vi "QuadRotor_Monitoring_LV3.vi"() -> ()   [LabVIEW 2015]
uses:
  <vilib>/Instr/_visa.llb/VISA Set IO Buffer Mask.ctl
  <vilib>/Instr/_visa.llb/VISA Configure Serial Port (Instr).vi
panel:
  out "GPS_Distance_T_G":dbl(slide) scale=0.0..200.0
  out "GPS_Distance__H_G":dbl(slide) scale=0.0..200.0
  out "GPS_Speed_Gaud":ext(knob) scale=0.0..80.0
  out "GPS_Distance_Transport":ext format="%#_3g"
  out "GPS_Distance_Home":ext format="%#_3g"
  out "GPS_LON_TRANSPORT":ext format="%#.7f"
  out "GPS_LAT_TRANSPORT":ext format="%#.7f"
  out "GPS_LON_HOME":ext format="%#.7f"
  out "GPS_LAT_HOME":ext format="%#.7f"
  out "Distance_R":dbl(slide)
  out "Distance_B":dbl(slide)
  out "Distance_F":dbl(slide) scale=0.0..800.0
  out "Distance_L":dbl(slide) scale=0.0..800.0
  out "MotorBackRf":dbl(slide) scale=1000.0..2000.0
  out "MotorBackLf":dbl(slide) scale=1000.0..2000.0
  out "MotorFrontRf":dbl(slide) scale=1000.0..2000.0
  out "MotorFrontLf":dbl(slide) scale=1000.0..2000.0
  in  "Lontitude_Transport":i32=1005738310
  in  "Latitude_Transport":i32=139458720
  in  "Lon_home":i32=1005748870
  in  "Lat_home":i32=139456050
  out "(GPS_numSat)":u16(slide) scale=0.0..20.0
  out "return count 2":u32
  out "Roob":i32
  out "Altitude_(Auto)":ext format="%#_3g"
  in  "Set_Altitude_(Auto)":dbl=2.5
  out "string":string
  out "Mode":ext format="%.2f"
  out "Altitude":dbl(slide) scale=0.0..20.0
  out "Altitude":ext format="%.2f"
  out "Yaw":dbl(knob) scale=-180.0..180.0
  out "Pitch":dbl(knob) scale=-90.0..90.0
  out "Roll":dbl(knob) scale=-90.0..90.0
  in  "Write to Quad":bool
  out "Header_58":u8
  out "GPS_LONGTITUDE":ext format="%#.7f"
  out "GPS_LATTITUDE":ext format="%#.7f"
  out "return count":u32
  in  "stop":bool
  in  "VISA Serial Data":refnum<visa-resource-name>
  # "Quad Rotor Monitoring and Control with GPS Waypoint"
  # "Data Write to Autonomous Quad Rotor (LAT 9 Point), (LON 10 Point) with Google Map tracking Navigator"
  # "Ex  13.8591411 = 138591411 , 100.5231704 = 1005231704 Using in integer  I32"
  # "9 Point"
  # "10 Point"
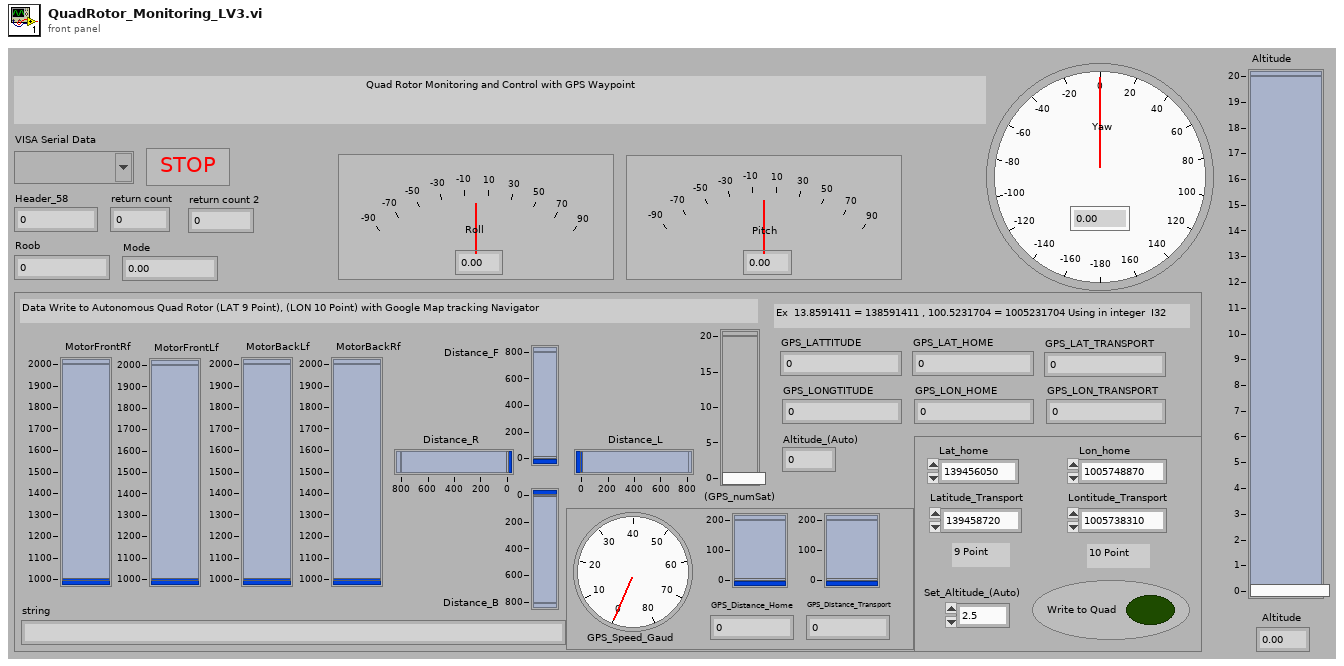
[diagram p1: front panel]
types:
  T1 = typedef "VISA Set IO Buffer Mask.ctl" = u16
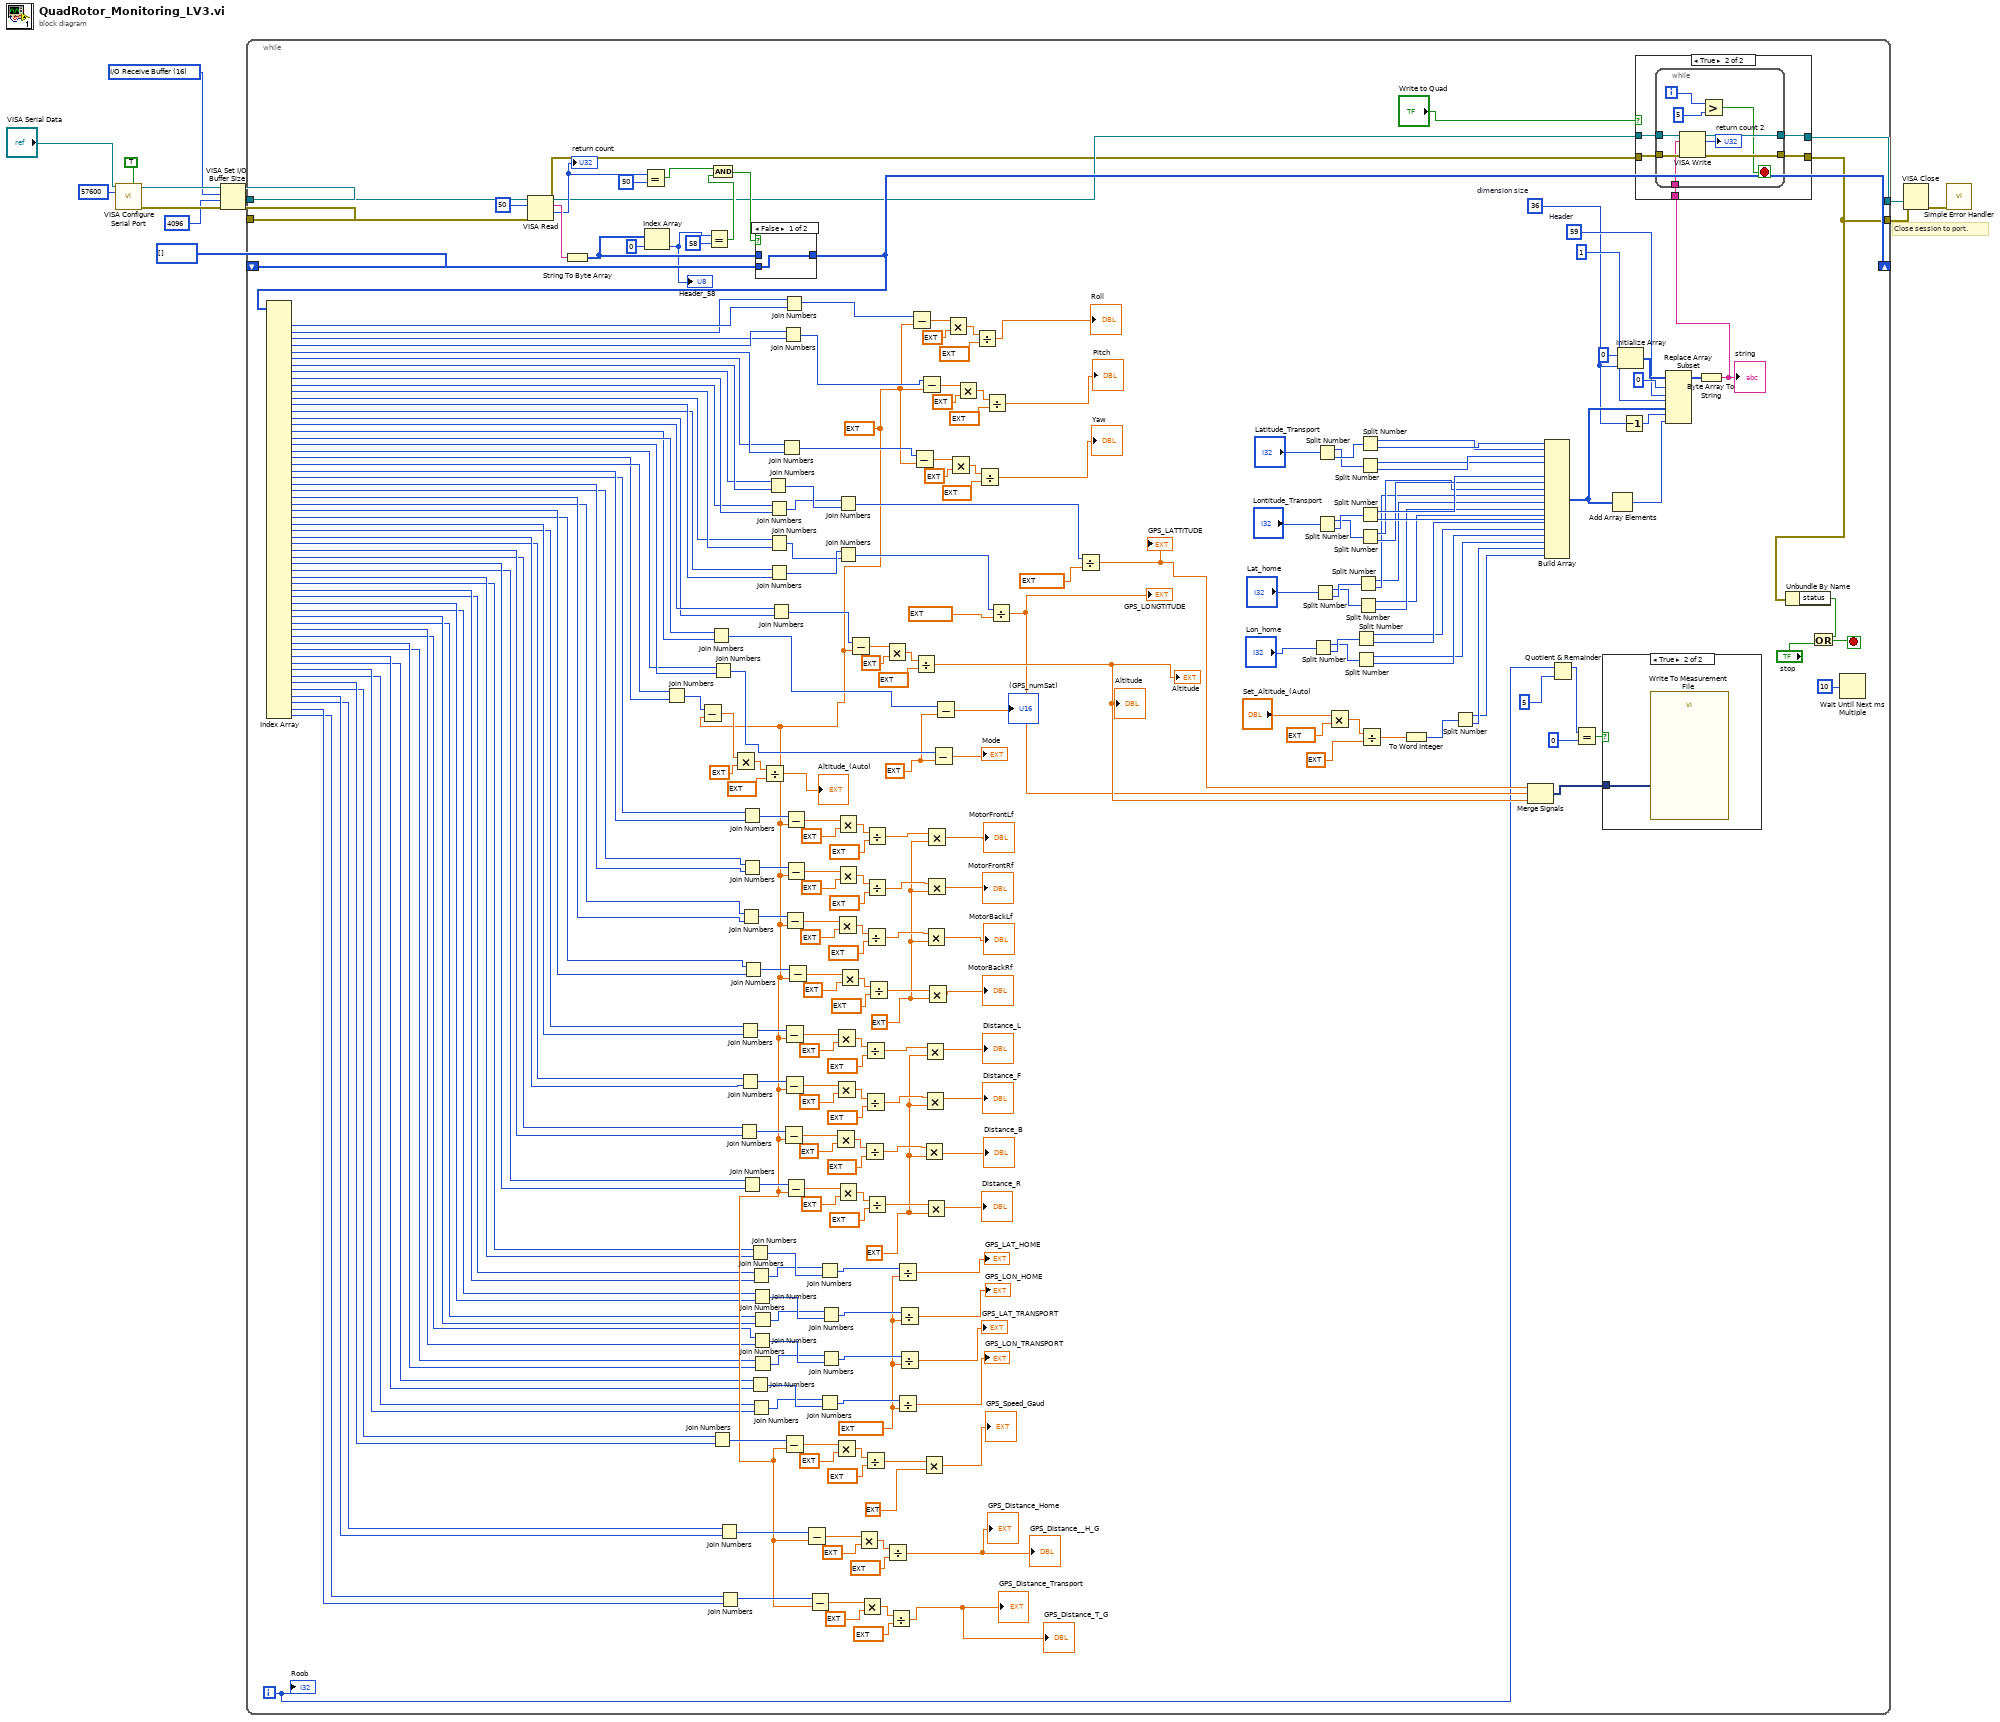
[diagram p0: block diagram]
diagram:
  w10 = T1 16 items=["I/O Receive Buffer"=16, "I/O Transmit Buffer"=32, "I/O Receive and Transmit Buffer"=48] ("Mask")
  # "Close session to port."
  n1 = call-poly "VISA Configure Serial Port"("VISA resource name"="VISA Serial Data", "Enable Termination\nChar (T)"=TRUE ("Enable Termination\nChar (T)"), "baud rate (9600)"=u32 57600) -> ("VISA resource name out"=w12:refnum<visa-resource-name>, "error out"=w11:errorcluster)  [unwired: 7 in, 4 out]
  n2 = VISA Set I/O Buffer Size(VISA resource name=w12, mask (16)=w10, size (4096)=u32 4096, error in (no error)=w11) -> (VISA resource name out=w8:refnum<visa-resource-name>, error out=w6:errorcluster)
  n3 = while {
    tunnel: [w247] -> w7
    tunnel: w8 -> [w288]
    tunnel: [w246] -> w5
    tunnel: w6 -> [w287]
    shift-right: [w257] -> _
    shift-left: u8[] [] ("unsigned byte array") -> [w258]
    i -> [w153]
    stop <- w291 stop-if-true
    w65 = ext 10000000.0 ("y")
    w86 = ext 10.0 ("y")
    w113 = ext 10.0 ("y")
    w168 = 36  # dimension size
    w215 = u8 59  # Header
    w160 = ext 255.0 ("y")
    w44 = ext 32767.0 ("y")
    n4 = VISA Read(VISA resource name=w288, byte count=u32 50, error in (no error)=w287) -> (VISA resource name out=w249:refnum<visa-resource-name>, read buffer=w261:string, return count=w254:u32, error out=w248:errorcluster)
    "return count" <- w254
    n5 = String To Byte Array(string=w261) -> (unsigned byte array=w259:u8[])
    n6 = Equal?(x=w254, y=u32 50) -> (x = y?=w252:bool)
    n7 = Index Array(array=w259, index=0) -> (element=w251:u8)
    "Header_58" <- w251
    n8 = Equal?(x=w251, y=u8 58) -> (x = y?=w256:bool)
    n9 = And(x=w252, y=w256) -> (x .and. y?=w255:bool)
    n10 = case shown="False" w255 {
      tunnel: w259 -> [_ w310]
      tunnel: [w309 w310] -> w257
      tunnel: w258 -> [w309 _]
      frame False {
      }
      frame True {
      }
    }
    n11 = Index Array(array=w257) -> (element #2=w281:u8, element #3=w280:u8, element #4=w278:u8, element #5=w279:u8, element #6=w285:u8, element #7=w284:u8, element #8=w283:u8, element #9=w282:u8, element #10=w242:u8, element #11=w241:u8, element #12=w238:u8, element #13=w237:u8, element #14=w236:u8, element #15=w235:u8, element #16=w226:u8, element #17=w232:u8, element #18=w224:u8, element #19=w225:u8, element #20=w223:u8, element #21=w222:u8, element #22=w179:u8, element #23=w180:u8, element #24=w129:u8, element #25=w128:u8, element #26=w127:u8, element #27=w126:u8, element #28=w125:u8, element #29=w124:u8, element #30=w123:u8, element #31=w122:u8, element #32=w43:u8, element #33=w42:u8, element #34=w41:u8, element #35=w40:u8, element #36=w39:u8, element #37=w38:u8, element #38=w37:u8, element #39=w36:u8, element #40=w35:u8, element #41=w34:u8, element #42=w33:u8, element #43=w32:u8, element #44=w31:u8, element #45=w30:u8, element #46=w29:u8, element #47=w28:u8, element #48=w27:u8, element #49=w26:u8, element #50=w25:u8, element #51=w24:u8, element #52=w23:u8, element #53=w22:u8, element #54=w21:u8, element #55=w20:u8, element #56=w19:u8, element #57=w18:u8, element #58=w17:u8, element #59=w16:u8, element #60=w15:u8, element #61=w14:u8)  [unwired: 61 in, 1 out]
    n12 = Join Numbers(hi=w180, lo=w179) -> ((hi.lo)=w178:u16)
    n13 = Subtract(x=w178, y=w44) -> (x-y=w174:ext)
    n14 = Join Numbers(hi=w225, lo=w224) -> ((hi.lo)=w159:u16)
    n15 = Join Numbers(hi=w18, lo=w19) -> ((hi.lo)=w60:u16)
    n16 = Join Numbers(hi=w222, lo=w223) -> ((hi.lo)=w163:u16)
    n17 = Join Numbers(hi=w16, lo=w17) -> ((hi.lo)=w52:u16)
    n18 = Join Numbers(hi=w14, lo=w15) -> ((hi.lo)=w47:u16)
    n19 = Multiply(x=w174, y=ext 100.0) -> (x*y=w176:ext)
    n20 = Join Numbers(hi=w38, lo=w39) -> ((hi.lo)=w96:u16)
    n21 = Join Numbers(hi=w42, lo=w43) -> ((hi.lo)=w106:u16)
    n22 = Join Numbers(hi=w40, lo=w41) -> ((hi.lo)=w101:u16)
    n23 = Join Numbers(hi=w124, lo=w125) -> ((hi.lo)=w135:u16)
    n24 = Join Numbers(hi=w128, lo=w129) -> ((hi.lo)=w145:u16)
    n25 = Join Numbers(hi=w126, lo=w127) -> ((hi.lo)=w140:u16)
    n26 = Join Numbers(hi=w36, lo=w37) -> ((hi.lo)=w91:u16)
    n27 = Join Numbers(hi=w122, lo=w123) -> ((hi.lo)=w130:u16)
    n28 = Join Numbers(hi=w34, lo=w35) -> ((hi.lo)=w81:u16)
    n29 = Join Numbers(hi=w22, lo=w23) -> ((hi.lo)=w72:u16)
    n30 = Join Numbers(hi=w32, lo=w33) -> ((hi.lo)=w80:u16)
    n31 = Join Numbers(hi=w20, lo=w21) -> ((hi.lo)=w71:u16)
    n32 = Join Numbers(hi=w30, lo=w31) -> ((hi.lo)=w78:u16)
    n33 = Join Numbers(hi=w26, lo=w27) -> ((hi.lo)=w75:u16)
    n34 = Join Numbers(hi=w28, lo=w29) -> ((hi.lo)=w77:u16)
    n35 = Join Numbers(hi=w24, lo=w25) -> ((hi.lo)=w74:u16)
    n36 = Divide(x=w176, y=ext 32767.0) -> (x/y=→"Altitude_(Auto)":ext)
    n37 = Join Numbers(hi=w282, lo=w283) -> ((hi.lo)=w240:u16)
    n38 = Join Numbers(hi=w241, lo=w242) -> ((hi.lo)=w239:u16)
    n39 = Join Numbers(hi=w237, lo=w238) -> ((hi.lo)=w220:u16)
    n40 = Join Numbers(hi=w235, lo=w236) -> ((hi.lo)=w221:u16)
    n41 = Join Numbers(hi=w232, lo=w226) -> ((hi.lo)=w227:u16)
    n42 = Join Numbers(hi=w284, lo=w285) -> ((hi.lo)=w267:u16)
    n43 = Join Numbers(hi=w279, lo=w278) -> ((hi.lo)=w262:u16)
    n44 = Subtract(x=w96, y=w44) -> (x-y=w99:ext)
    n45 = Join Numbers(hi=w280, lo=w281) -> ((hi.lo)=w276:u16)
    n46 = Subtract(x=w106, y=w44) -> (x-y=w109:ext)
    n47 = Subtract(x=w101, y=w44) -> (x-y=w104:ext)
    n48 = Subtract(x=w60, y=w44) -> (x-y=w63:ext)
    n49 = Subtract(x=w135, y=w44) -> (x-y=w138:ext)
    n50 = Subtract(x=w145, y=w44) -> (x-y=w148:ext)
    n51 = Subtract(x=w140, y=w44) -> (x-y=w143:ext)
    n52 = Subtract(x=w91, y=w44) -> (x-y=w94:ext)
    n53 = Subtract(x=w130, y=w44) -> (x-y=w133:ext)
    n54 = Subtract(x=w52, y=w44) -> (x-y=w55:ext)
    n55 = Subtract(x=w47, y=w44) -> (x-y=w50:ext)
    n56 = Join Numbers(hi=w80, lo=w81) -> ((hi.lo)=w79:u32)
    n57 = Join Numbers(hi=w71, lo=w72) -> ((hi.lo)=w70:u32)
    n58 = Join Numbers(hi=w77, lo=w78) -> ((hi.lo)=w76:u32)
    n59 = Join Numbers(hi=w74, lo=w75) -> ((hi.lo)=w73:u32)
    n60 = Multiply(x=w99, y=ext 100.0) -> (x*y=w100:ext)
    n61 = Multiply(x=w109, y=ext 100.0) -> (x*y=w110:ext)
    n62 = Multiply(x=w104, y=ext 100.0) -> (x*y=w105:ext)
    n63 = Multiply(x=w63, y=ext 100.0) -> (x*y=w64:ext)
    n64 = Multiply(x=w138, y=ext 185.0) -> (x*y=w139:ext)
    n65 = Join Numbers(hi=w239, lo=w240) -> ((hi.lo)=w244:u32)
    n66 = Join Numbers(hi=w221, lo=w220) -> ((hi.lo)=w234:u32)
    n67 = Multiply(x=w148, y=ext 185.0) -> (x*y=w149:ext)
    n68 = Multiply(x=w143, y=ext 185.0) -> (x*y=w144:ext)
    n69 = Multiply(x=w94, y=ext 100.0) -> (x*y=w95:ext)
    n70 = Multiply(x=w133, y=ext 185.0) -> (x*y=w134:ext)
    n71 = Subtract(x=w227, y=w44) -> (x-y=w231:ext)
    n72 = Multiply(x=w55, y=ext 200.0) -> (x*y=w56:ext)
    n73 = Multiply(x=w50, y=ext 200.0) -> (x*y=w51:ext)
    n74 = Divide(x=w100, y=ext 32767.0) -> (x/y=w89:ext)
    n75 = Divide(x=w110, y=ext 32767.0) -> (x/y=w87:ext)
    n76 = Divide(x=w105, y=ext 32767.0) -> (x/y=w88:ext)
    n77 = Divide(x=w64, y=ext 32767.0) -> (x/y=w59:ext)
    n78 = Divide(x=w139, y=ext 32767.0) -> (x/y=w116:ext)
    n79 = Divide(x=w149, y=ext 32767.0) -> (x/y=w114:ext)
    n80 = Divide(x=w144, y=ext 32767.0) -> (x/y=w115:ext)
    n81 = Divide(x=w95, y=ext 32767.0) -> (x/y=w90:ext)
    n82 = Divide(x=w134, y=ext 32767.0) -> (x/y=w121:ext)
    n83 = Multiply(x=w231, y=ext 100.0) -> (x*y=w229:ext)
    n84 = Divide(x=w56, y=ext 32767.0) -> (x/y=→"GPS_Distance_Home" →"GPS_Distance__H_G":ext)
    n85 = Divide(x=w51, y=ext 32767.0) -> (x/y=→"GPS_Distance_Transport" →"GPS_Distance_T_G":ext)
    n86 = Divide(x=w79, y=w65) -> (x/y=→"GPS_LAT_HOME":ext)
    n87 = Divide(x=w70, y=w65) -> (x/y=→"GPS_LON_TRANSPORT":ext)
    n88 = Divide(x=w76, y=w65) -> (x/y=→"GPS_LON_HOME":ext)
    n89 = Divide(x=w73, y=w65) -> (x/y=→"GPS_LAT_TRANSPORT":ext)
    n90 = Subtract(x=w276, y=w44) -> (x-y=w275:ext)
    n91 = Subtract(x=w267, y=w44) -> (x-y=w271:ext)
    n92 = Divide(x=w229, y=ext 32767.0) -> (x/y=w158:ext)
    "Altitude" <- w158
    "Altitude" <- w158
    n93 = Subtract(x=w262, y=w44) -> (x-y=w266:ext)
    n94 = Multiply(x=w89, y=w86) -> (x*y=→"Distance_B":ext)
    n95 = Multiply(x=w59, y=ext 10.0) -> (x*y=→"GPS_Speed_Gaud":ext)
    n96 = Multiply(x=w87, y=w86) -> (x*y=→"Distance_L":ext)
    n97 = Multiply(x=w88, y=w86) -> (x*y=→"Distance_F":ext)
    n98 = Multiply(x=w116, y=w113) -> (x*y=→"MotorBackLf":ext)
    n99 = Multiply(x=w90, y=w86) -> (x*y=→"Distance_R":ext)
    n100 = Multiply(x=w114, y=w113) -> (x*y=→"MotorFrontLf":ext)
    n101 = Multiply(x=w115, y=w113) -> (x*y=→"MotorFrontRf":ext)
    n102 = Multiply(x=w121, y=w113) -> (x*y=→"MotorBackRf":ext)
    n103 = Subtract(x=w163, y=w160) -> (x-y=→"Mode":ext)
    n104 = Subtract(x=w159, y=w160) -> (x-y=→"(GPS_numSat)":ext)
    n105 = Multiply(x=w275, y=ext 180.0) -> (x*y=w273:ext)
    n106 = Multiply(x=w271, y=ext 180.0) -> (x*y=w269:ext)
    n107 = Multiply(x=w266, y=ext 180.0) -> (x*y=w264:ext)
    n108 = Divide(x=w273, y=ext 32767.0) -> (x/y=→"Roll":ext)
    n109 = Divide(x=w269, y=ext 32767.0) -> (x/y=→"Yaw":ext)
    n110 = Divide(x=w264, y=ext 32767.0) -> (x/y=→"Pitch":ext)
    n111 = Divide(x=w234, y=ext 10000000.0) -> (x/y=w157:ext)
    "GPS_LONGTITUDE" <- w157
    n112 = Divide(x=w244, y=ext 10000000.0) -> (x/y=w156:ext)
    "GPS_LATTITUDE" <- w156
    n113 = Split Number(x="Lon_home") -> (hi(x)=w208:u16, lo(x)=w209:u16)
    n114 = Split Number(x="Lat_home") -> (hi(x)=w210:u16, lo(x)=w211:u16)
    n115 = Split Number(x="Lontitude_Transport") -> (hi(x)=w212:u16, lo(x)=w213:u16)
    n116 = Split Number(x="Latitude_Transport") -> (hi(x)=w190:u16, lo(x)=w191:u16)
    n117 = Multiply(x="Set_Altitude_(Auto)", y=ext 32767.0) -> (x*y=w183:ext)
    n118 = Split Number(x=w209) -> (hi(x)=w194:u8, lo(x)=w195:u8)
    n119 = Split Number(x=w208) -> (hi(x)=w192:u8, lo(x)=w193:u8)
    n120 = Split Number(x=w211) -> (hi(x)=w198:u8, lo(x)=w199:u8)
    n121 = Split Number(x=w210) -> (hi(x)=w196:u8, lo(x)=w197:u8)
    n122 = Split Number(x=w213) -> (hi(x)=w202:u8, lo(x)=w203:u8)
    n123 = Split Number(x=w212) -> (hi(x)=w200:u8, lo(x)=w201:u8)
    n124 = Split Number(x=w191) -> (hi(x)=w206:u8, lo(x)=w207:u8)
    n125 = Split Number(x=w190) -> (hi(x)=w204:u8, lo(x)=w205:u8)
    n126 = Divide(x=w183, y=ext 100.0) -> (x/y=w181:ext)
    n127 = To Word Integer(number=w181) -> (16bit integer=w184:i16)
    n128 = Split Number(x=w184) -> (hi(x)=w185:u8, lo(x)=w186:u8)
    n129 = Merge Signals(w156, w157, w158) -> (w155:dynamicdata)
    n130 = Build Array(w207, w206, w205, w204, w203, w202, w201, w200, w199, w198, w197, w196, w195, w194, w193, w192, w186, w185) -> (w171:u8[])
    n131 = Quotient & Remainder(x=w153, y=u32 5) -> (x-y*floor(x/y)=w150:u32)  [unwired: 1 out]
    n132 = Equal?(x=w150, y=u32 0) -> (x = y?=w152:bool)
    n133 = case shown="True" w152 {
      tunnel: w155 -> [_ w292]
      frame False {
      }
      frame True {
        n134 = call "Write To Measurement File"("Signals"=w292) -> ()  [unwired: 16 in, 3 out]
      }
    }
    n135 = Add Array Elements(numeric array=w171) -> (sum=w170:u8)
    n136 = Initialize Array(u8 0, w168) -> (w219:u8[])
    n137 = Decrement(x=w168) -> (x-1=w169:i32)
    n138 = Replace Array Subset(array=w219, new element #1=w215, index #1=0 ("index"), new element #2=w171, index #2=1 ("index"), new element #3=w170, index #3=w169) -> (w214:u8[])
    n139 = Byte Array To String(unsigned byte array=w214) -> (string=w189:string)
    "string" <- w189
    n140 = case shown="True" "Write to Quad" {
      tunnel: w249 -> [w293 w299]
      tunnel: w248 -> [w294 w296]
      tunnel: [w293 w298] -> w247
      tunnel: [w294 w297] -> w246
      tunnel: w189 -> [_ w295]
      frame False {
      }
      frame True {
        n141 = while {
          tunnel: w299 -> [w308]
          tunnel: [w307] -> w298
          tunnel: [w306] -> w297
          tunnel: w296 -> [w305]
          tunnel: w295 -> [w304]
          i -> [w302]
          stop <- w300 stop-if-true
          n142 = VISA Write(VISA resource name=w308, write buffer=w304, error in (no error)=w305) -> (VISA resource name out=w307:refnum<visa-resource-name>, return count=→"return count 2":u32, error out=w306:errorcluster)
          n143 = Greater?(x=w302, y=5) -> (0:w300:bool)
        }
      }
    }
    n144 = Unbundle By Name(w246) -> ("status"=w289:bool)
    n145 = Or(x=w289, y="stop") -> (x .or. y?=w291:bool)
    n146 = Wait Until Next ms Multiple(millisecond multiple=u32 10) -> ()  [unwired: 1 out]
    "Roob" <- w153
  }
  n147 = VISA Close(VISA resource name=w7, error in (no error)=w5) -> (error out=w9:errorcluster)
  n148 = call <vilib>:"Simple Error Handler.vi"("error in (no error)"=w9) -> ()  [unwired: 1 in, 8 out]
